vi "IO_CloseDevice.vi"(4 "error in":errorcluster caption="错误输入", 7 "hDevice":u32) -> (0 "error out":errorcluster caption="错误输出", 1 "hDevictOut":u32, 3 "返回值":i32)   [LabVIEW 2013]
uses:
  FY2400P.dll
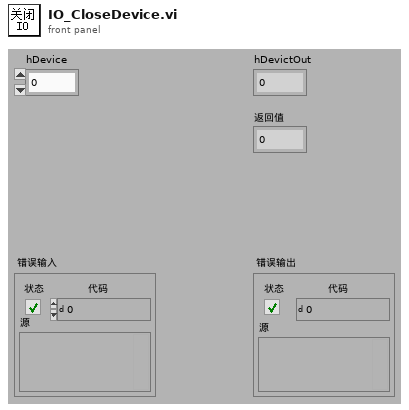
[diagram p1: front panel]
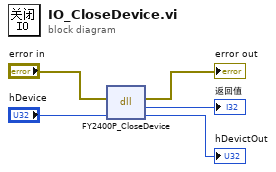
[diagram p0: block diagram]
diagram:
  n1 = dll-call lib="PTH1\\abs E桌面休眠电流方案休眠电流源码20181130\nInstrumentIOFY2400P.dll" fn="FY2400P_CloseDevice"(error in="error in", "hDevice"="hDevice") -> (error out=→"error out":errorcluster, "返回类型"=→"返回值":i32, "hDevice"=→"hDevictOut":u32)  [unwired: 2 in, 1 out]
